vi "find element with id.vi"(8 "error in (no error)":errorcluster, 10 "id":string, 11 "IDable Array in":refnum<class "IDable.lvclass">[](array[class])) -> (0 "error out":errorcluster, 2 "index":i32)   [LabVIEW 2017, in "ID API.lvclass"]
uses:
  ID API.lvclass
  IDable/IDable.lvclass
  IDable/IDable.lvclass/IDable.ctl
  IDable/Read id.vi
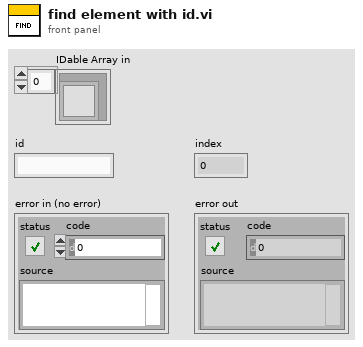
[diagram p1: front panel]
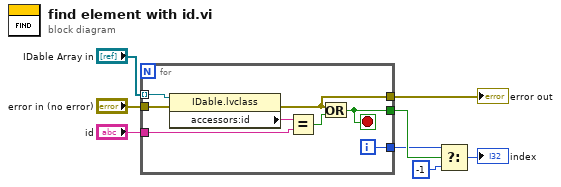
[diagram p0: block diagram]
diagram:
  n1 = for {
    tunnel: "IDable Array in" -> [w16] mode=indexing
    tunnel: "id" -> [w14]
    tunnel: [w13] -> w5
    tunnel: [w10] -> w6
    tunnel: "error in (no error)" -> [w11]
    tunnel: [w9] -> w1
    i -> [w13]
    stop <- w10 stop-if-true
    n2 = property class="IDable.lvclass"(reference=w16, error in=w11) -> (error out=w9:errorcluster, "accessors:id"=w15:string)  [unwired: 1 out]
    n3 = Equal?(x=w15, y=w14) -> (x = y?=w12:bool)
    n4 = Or(x=w9, y=w12) -> (x .or. y?=w10:bool)
  }
  "error out" <- w1
  n5 = Select(t=w5, s=w6, f=-1) -> (s? t:f=→"index":i32)
